vi "SR04 working.vi"() -> ()   [LabVIEW 2017, in "LIFA Ultrasonic Distance.lvlib"]
uses:
  LIFA Ultrasonic Distance LV9/LIFA Ultrasonic Distance.lvlib
  <vilib>/LabVIEW Interface for Arduino/Type Defs/Board Type.ctl
  LIFA Ultrasonic Distance LV9/Get Distance/HC-SR04 Get Distance.vi
  <vilib>/LabVIEW Interface for Arduino/LabVIEW Interface for Arduino.lvlib
panel:
  out "Distance (cm)":dbl
  in  "stop":bool
  # "1.  Upload the provided LIFA firmware.\n\n2.  If using a board other than the Arduino UNO, change the parameters for Init.vi on the block diagram.\n\n3.  Wire the signal pin of the sensor to Arduino pin 8. \n\n4.  Run the VI."
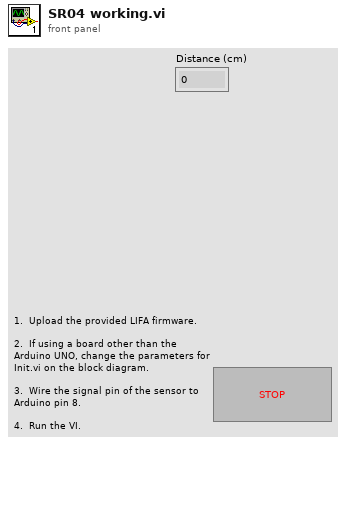
[diagram p1: front panel]
types:
  T1 = typedef "LabVIEW Interface for Arduino.lvlib/Board Type.ctl" = enum16{"Uno", "Dimuelanove w/Atmega 328", "Mega 2560"}
  T2 = typedef "LabVIEW Interface for Arduino.lvlib/Arduino Resource.ctl" = cluster{"VISA resource":refnum<visa-resource-name>, "Board Type":T1, "Connection Type":enum8{"USB / Serial"}, "Bytes Per Packet (15)":u8}
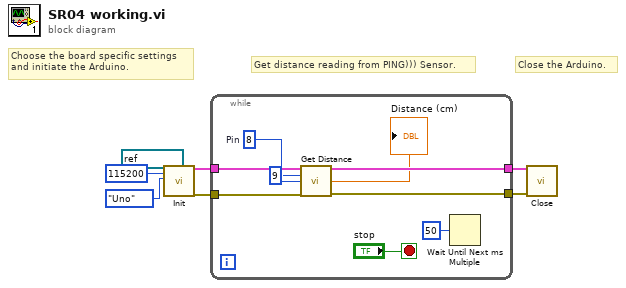
[diagram p0: block diagram]
diagram:
  # "Close the Arduino."
  # "Get distance reading from PING))) Sensor."
  # "Choose the board specific settings\nand initiate the Arduino."
  n1 = call <vilib>:"Init.vi"("VISA resource"=refnum<visa-resource-name> "COM4", "Baud Rate (115200)"=u32 115200, "Board Type (Uno)"=Board_Type."Uno") -> ("Arduino Resource"=w7:T2, "error out"=w6:errorcluster)  [unwired: 15 in]
  n2 = while {
    tunnel: w7 -> [w15]
    tunnel: w6 -> [w14]
    tunnel: [w12] -> w4
    tunnel: [w11] -> w5
    stop <- "stop" stop-if-true
    w13 = u8 8  # Pin
    n3 = call-poly "Get Distance.vi"("Arduino Resource"=w15, "Trigger Pin"=u8 9, "Signal Pin"=w13, "error in (no error)"=w14) -> ("Arduino Resource"=w11:T2, "Distance (cm)"=→"Distance (cm)":dbl, "error out"=w12:errorcluster)  [unwired: 9 in]
    n4 = Wait Until Next ms Multiple(millisecond multiple=u32 50) -> ()  [unwired: 1 out]
  }
  n5 = call <vilib>:"Close.vi"("Arduino Resource"=w5, "error in"=w4) -> ()  [unwired: 13 in, 1 out]
